vi "Read From VS Parameter FIFO.vi"(8 "Error In":errorcluster, 11 "Async State Vars":T1) -> (0 "Error Out":errorcluster, 1 "Parameter FIFO empty?":bool, 3 "Async State Vars out":T1)   [LabVIEW 2017, in "Waveform-Processing-Custom-Device Engine.lvlib"]
uses:
  Waveform-Processing-Custom-Device Engine.lvlib
  Types/AsyncStateVariables.ctl
  <vilib>/NI Veristand/Custom Device Waveform API/Single Waveform Read (DBL)/Single Waveform Read (DBL).lvclass
  <vilib>/NI Veristand/Custom Device Waveform API/Single Waveform Write (DBL)/Single Waveform Write (DBL).lvclass
  <vilib>/NI Veristand/Custom Device API/Waveform Data Reference.ctl
  Types/New Async FIFOs.ctl
  <vilib>/NI/NIVS Inline Async API/_Data Access Engine/Data Access Engine/Types/Write.DVR.ctl
  <vilib>/NI/NIVS Inline Async API/_Data Access Engine/Access Type Classes/Write/Write.lvclass
  <vilib>/NI/NIVS Inline Async API/_Data Access Engine/Data Access Engine/Types/Read.DVR.ctl
  <vilib>/NI/NIVS Inline Async API/_Data Access Engine/Access Type Classes/Read/Read.lvclass
  <vilib>/NI/NIVS Inline Async API/_Data Access Engine/Access Type Classes/Read/Read.lvclass/Read.ctl
  <vilib>/NI/NIVS Inline Async API/_Data Access Engine/Data Access Engine/Methods/Read.Data.vi
  <vilib>/NI/NIVS Inline Async API/_Data Access Engine/Access Type Classes/Read/Read.ProcessData.vi
  <vilib>/NI/NIVS Inline Async API/_Data Access Engine/Data Access Engine/Data Access Engine.lvclass
  <vilib>/NI Veristand/Custom Device API/Custom Device API.lvlib
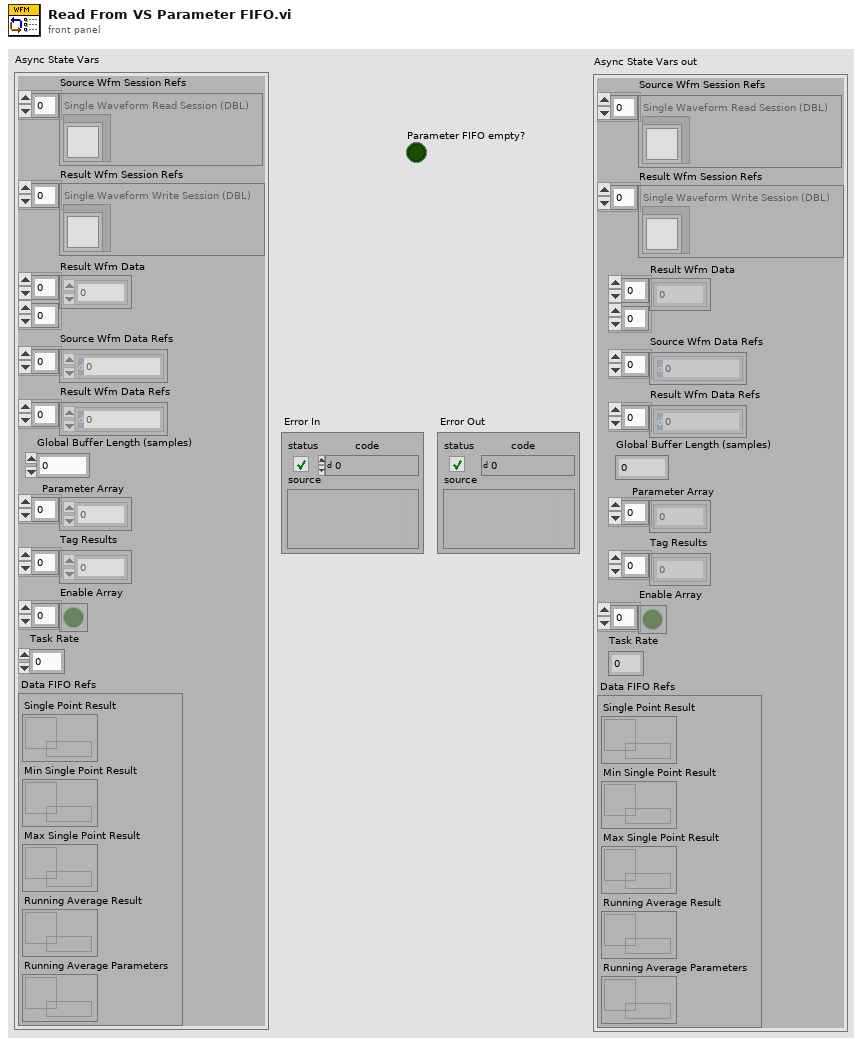
[diagram p1: front panel]
types:
  T1 = typedef "Waveform-Processing-Custom-Device Engine.lvlib/AsyncStateVariables.ctl" = cluster{"Source Wfm Session Refs":refnum<class "Single Waveform Read (DBL).lvclass">[], "Result Wfm Session Refs":refnum<class "Single Waveform Write (DBL).lvclass">[], "Result Wfm Data":dbl[][], "Source Wfm Data Refs":T2[], "Result Wfm Data Refs":T2[], "Global Buffer Length (samples)":dbl, "Parameter Array":dbl[], "Tag Results":dbl[], "Enable Array":bool[], "Task Rate":dbl, "Data FIFO Refs":T3}
  T2 = typedef "Custom Device API.lvlib/Waveform Data Reference.ctl" = i32
  T3 = typedef "Waveform-Processing-Custom-Device Engine.lvlib/New Async FIFOs.ctl" = cluster{"Single Point Result":T4, "Running Average Result":T4, "Running Average Parameters":T5, "Min Single Point Result":T4, "Max Single Point Result ":T4}
  T4 = typedef "Data Access Engine.lvlib/Data Access Engine.lvclass/Write.DVR.ctl" = refnum<data-value>
  T5 = typedef "Data Access Engine.lvlib/Data Access Engine.lvclass/Read.DVR.ctl" = refnum<data-value>
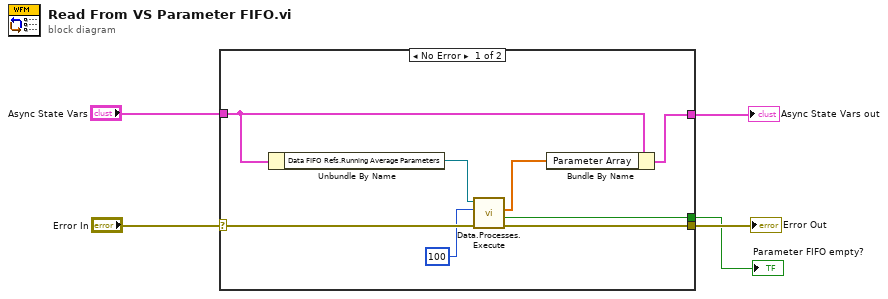
[diagram p0: block diagram]
diagram:
  n1 = case shown="No Error" "Error In" {
    selector: "Error In" -> [w11 w15]
    tunnel: [w7 w15] -> w4
    tunnel: "Async State Vars" -> [w13 w14]
    tunnel: [w12 w14] -> w2
    tunnel: [w6 _] -> w1
    frame No Error {
      n2 = Unbundle By Name(w13) -> ("Data FIFO Refs.Running Average Parameters"=w10:T5)
      n3 = call-poly <vilib>:"Data.Processes.Execute.vi"("error in"=w11, "timeout ms"=100, "Ref"=w10) -> ("error out"=w7:errorcluster, "Timeout?"=w6:bool, "Values"=w9:dbl[])  [unwired: 6 in]
      n4 = Bundle By Name(cluster=w13, "Parameter Array"=w9) -> (w12:T1)
    }
    frame Error {
    }
  }
  "Error Out" <- w4
  "Async State Vars out" <- w2
  "Parameter FIFO empty?" <- w1
